vi "Transform2d_Inverse.vi"(11 "inTRANSFORM":T1={"TRANSLATION"={"X"=0.0, "Y"=0.0}, "ROTATION"={"VALUE"=0.0, "COS"=1.0, "SIN"=0.0}, "xF"=FALSE} {"ROTATION"."SIN" format="%13.4f"; "ROTATION"."COS" format="%13.4f"; "ROTATION"."VALUE" format="%13.4f"; "TRANSLATION"."Y" format="%14.3f"; "TRANSLATION"."X" format="%14.3f"}) -> (3 "TRANSFORM":T1 {"ROTATION"."SIN" format="%13.4f"; "ROTATION"."COS" format="%13.4f"; "ROTATION"."VALUE" format="%13.4f"; "TRANSLATION"."Y" format="%14.3f"; "TRANSLATION"."X" format="%14.3f"})   [LabVIEW 2019, in "Trajectory_Library.lvlib"]
doc: "Invert the transformation. This is useful for undoing a transformation.\n\nParameters:\n - IN TRANSFORM - This TRANSFORM data structure\n\nResults:\n - OUT TRANSFORM - The inverted transformation."
uses:
  Trajectory_Library.lvlib
  TypeDef/TRANSLATION2D.ctl
  TypeDef/ROTATION2D.ctl
  TypeDef/TRANSFORM2D.ctl
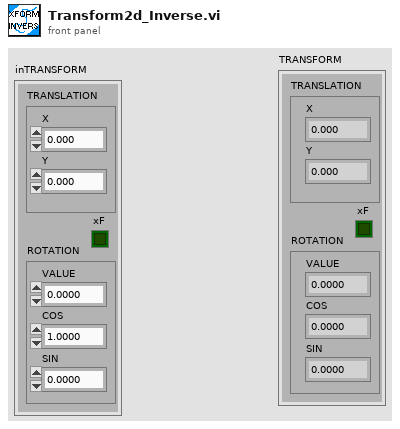
[diagram p1: front panel]
types:
  T1 = typedef "Trajectory_Library.lvlib/TRANSFORM2D.ctl" = cluster{"TRANSLATION":T2, "ROTATION":T3, "xF":bool}
  T2 = typedef "Trajectory_Library.lvlib/TRANSLATION2D.ctl" = cluster{"X":dbl, "Y":dbl}
  T3 = typedef "Trajectory_Library.lvlib/ROTATION2D.ctl" = cluster{"VALUE":dbl, "COS":dbl, "SIN":dbl}
  T4 = typedef "WPILib_Math.lvlib/TRANSFORM2D.ctl" = cluster{"TRANSLATION":T5, "ROTATION":T6, "xF":bool}
  T5 = typedef "WPILib_Math.lvlib/TRANSLATION2D.ctl" = cluster{"X":dbl, "Y":dbl}
  T6 = typedef "WPILib_Math.lvlib/ROTATION2D.ctl" = cluster{"VALUE":dbl, "COS":dbl, "SIN":dbl}
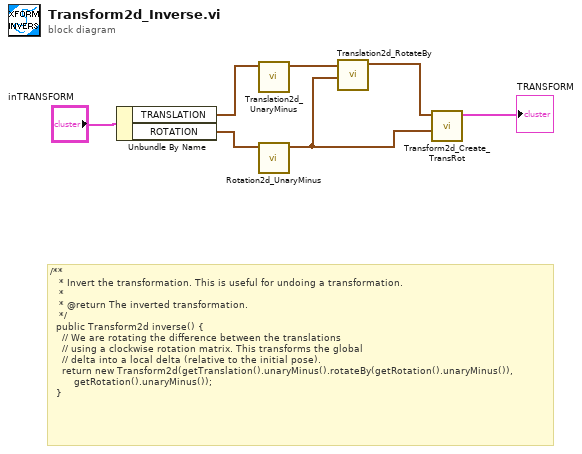
[diagram p0: block diagram]
diagram:
  # "/**\n   * Invert the transformation. This is useful for undoing a transformation.\n   *\n   * @return The inverted transformation.\n   */\n  public Transform2d inverse() {\n    // We are rotating the difference between the translations\n    // using a clockwise rotation matrix. This transforms the global\n    // delta into a local delta (relative to the initial pose).\n    return new Transform2d(getTranslation().unaryMinus().rotateBy(getRotation().unaryMinus()),\n        getRotation().unaryMinus());\n  }"
  n1 = Unbundle By Name("inTRANSFORM") -> ("TRANSLATION"=w5:T2, "ROTATION"=w4:T3)
  n2 = call "Translation2d_UnaryMinus.vi"("In Translation"=w5) -> ("Out Translation"=w3:T2)  [unwired: 10 in]
  n3 = call "Rotation2d_UnaryMinus.vi"("in ROTATION"=w4) -> ("out ROTATION"=w1:T3)  [unwired: 10 in]
  n4 = call "Translation2d_RotateBy.vi"("other Rotation"=w1, "In Translation"=w3) -> ("Out Translation"=w2:T2)  [unwired: 9 in]
  n5 = call "Transform2d_Create_TransRot.vi"("ROTATION"=w1, "TRANSLATION"=w2) -> ("TRANSFORM"=→"TRANSFORM":T4)  [unwired: 9 in]
